vi "Set timeline Y-axis.vi"(8 "error in (no error)":errorcluster, 10 "Data In":T2, 11 "Timeline Graph in":T1) -> (0 "error out":errorcluster, 3 "Timeline Graph out":T1)   [LabVIEW 2017, in "XGrapher.xctl"]
uses:
  XGrapher.xctl
  Data 1.ctl
  Typedefs/Xctrl-Data array.ctl
  Typedefs/Xcrtl-Data format definition.ctl
  Typedefs/Xctl-XY data type definition.ctl
  Typedefs/Xctrl-ROI type enum.ctl
  Typedefs/Xctrl-Timeline graph ref.ctl
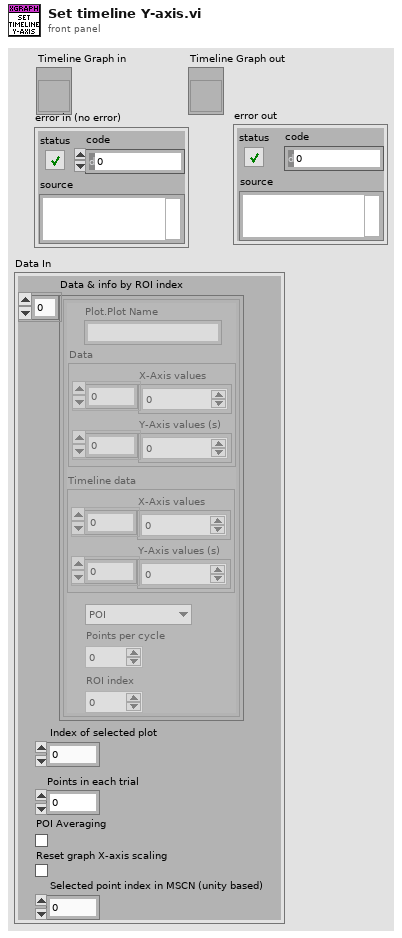
[diagram p1: front panel]
types:
  T1 = typedef "XGrapher.xctl/Xctrl-Timeline graph ref.ctl" = refnum<vi>
  T2 = typedef "XGrapher.xctl/Data 1.ctl" = cluster{"Data & info by ROI index":T3, "Index of selected plot":u16, "Points in each trial":i32, "POI Averaging":bool, "Reset graph X-axis scaling":bool, "Selected point index in MSCN (unity based)":u16}
  T3 = typedef "Xctrl-Data array.ctl" = T4[]
  T4 = typedef "XGrapher.xctl/Xcrtl-Data format definition.ctl" = cluster{"Plot.Plot Name":string, "Data":T5, "Timeline data":T5, "Type":T6, "Points per cycle":u16, "ROI index":u16}
  T5 = typedef "XGrapher.xctl/Xctl-XY data type definition.ctl" = cluster{"X-Axis values":sgl[], "Y-Axis values (s)":sgl[]}
  T6 = typedef "Xctrl-ROI type enum.ctl" = enum16{"POI", "Mini-scan", "Group"}
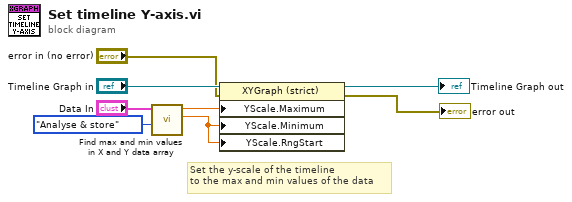
[diagram p0: block diagram]
diagram:
  # "Set the y-scale of the timeline \nto the max and min values of the data"
  n1 = call "Find max and min values in X and Y data array.vi"("Function"=enum16{"Analyse & store", "Read stored values"}."Analyse & store", "Data In"="Data In") -> ("Min intensity among all datasets"=w4:dbl, "Max intensity among all datasets"=w5:dbl)  [unwired: 5 in, 3 out]
  n2 = property on="Property Node" class="XYGraph (strict)"(reference="Timeline Graph in", error in="error in (no error)", "YScale.Maximum"=w5, "YScale.Minimum"=w4, "YScale.RngStart"=w4) -> (reference out=→"Timeline Graph out":T1, error out=→"error out":errorcluster)
